vi "Wire Two Objects.vi"(8 "error in (no error)":errorcluster, 10 "input cluster":T1, 11 "Data Cluster in":T2) -> (0 "error out":errorcluster, 2 "result":string, 3 "Data Cluster out":T2)   [LabVIEW 2025, in "Scripting Server.lvlib"]
uses:
  Scripting Server.lvlib
  Module Data--cluster.ctl
  Connect Objects Argument--cluster.ctl
  Connect Objects (Reply Payload)--cluster.ctl
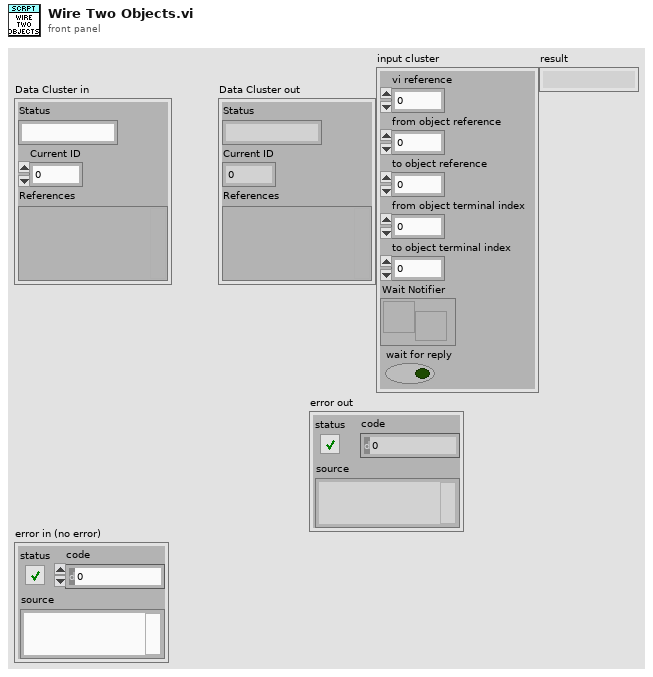
[diagram p1: front panel]
types:
  T1 = typedef "Scripting Server.lvlib/Connect Objects Argument--cluster.ctl" = cluster{"vi reference":i32, "from object reference":i32, "to object reference":i32, "from object terminal index":i32, "to object terminal index":i32, "Wait Notifier":refnum<notifier>, "wait for reply":bool}
  T2 = typedef "Scripting Server.lvlib/Module Data--cluster.ctl" = cluster{"Status":string, "Current ID":i32, "References":variant}
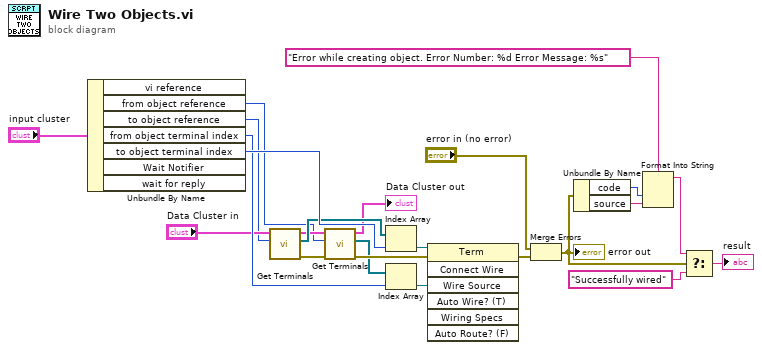
[diagram p0: block diagram]
diagram:
  n1 = Unbundle By Name("input cluster") -> ("from object reference"=w2:i32, "to object reference"=w6:i32, "from object terminal index"=w15:i32, "to object terminal index"=w19:i32)  [unwired: 3 out]
  n2 = call "Get Terminals.vi"("to object reference"=w6, "Data Cluster in"="Data Cluster in") -> ("error out"=w8:errorcluster, "Terms[]"=w14:refnum<vi>[], "Data Cluster out"=w4:T2)  [unwired: 7 in]
  n3 = call "Get Terminals.vi"("error in (no error)"=w8, "to object reference"=w2, "Data Cluster in"=w4) -> ("error out"=w5:errorcluster, "Terms[]"=w1:refnum<vi>[], "Data Cluster out"=→"Data Cluster out":T2)  [unwired: 6 in]
  n4 = Index Array(array=w14, index=w19) -> (element=w18:refnum<vi>)
  n5 = Index Array(array=w1, index=w15) -> (element=w20:refnum<vi>)
  n6 = invoke class="Term" method="Connect Wire"(reference=w18, error in=w5, "Wire Source"=w20) -> (error out=w23:errorcluster)  [unwired: 4 in, 6 out]
  n7 = Merge Errors("error in (no error)", w23) -> (w11:errorcluster)
  "error out" <- w11
  n8 = Unbundle By Name(w11) -> ("code"=w12:i32, "source"=w13:string)
  n9 = Format Into String(format string="Error while creating object. Error Number: %d Error Message: %s" ("f"), w12, w13) -> (resulting string=w9:string)  [unwired: 2 in, 1 out]
  n10 = Select(t=w9, s=w11, f="Successfully wired") -> (s? t:f=→"result":string)
